vi "Brickbreaker.vi"() -> ()   [LabVIEW 2023]
uses:
  <vilib>/Utility/miscctls.llb/LVPositionTypeDef.ctl
panel:
  out "Brick":bool=TRUE
  out "Top":bool
  out "exit?":bool
  in  "STOP":bool
  out "BarPosition":T1
  out "BallPosition":T1
  out "Step":T1
  out "Score":i32
  out "Bar":bool
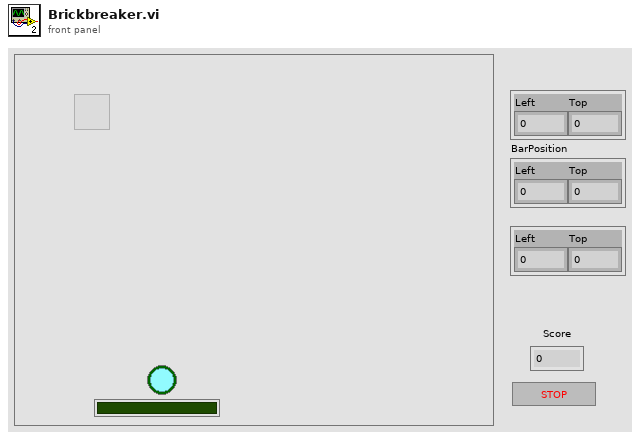
[diagram p1: front panel]
types:
  T1 = typedef "LVPositionTypeDef.ctl" = cluster{"Left":i32, "Top":i32}
  T2 = cluster{"BallPosition":T1, "Step":T1, "Score":i32, "BarPosition":T1, "BrickPosition":T1}
  T3 = typedef "eventvkey.ctl" = enum16{"ASCII", "Enter", "Return", "Shift", "Ctrl", "Alt", "Cmd", "Opt", "Caps", "NumLock", "Clear", "Break", "Up", "Down", "Left", "Right", "Insert", "Delete", "Home", "End", "PageUp", "PageDown", "Escape", "Help", "Pause", "ScrollLock", "F1", "F2", "F3", "F4", "F5", "F6", "F7", "F8", "F9", "F10", "F11", "F12", "F13", "F14", "F15", "F16", "F17", "F18", "F19", "F20", "F21", "F22", "F23", "F24", "Play", "VolumeUp", "VolumeDown", "Mute", "Two Byte Char"}
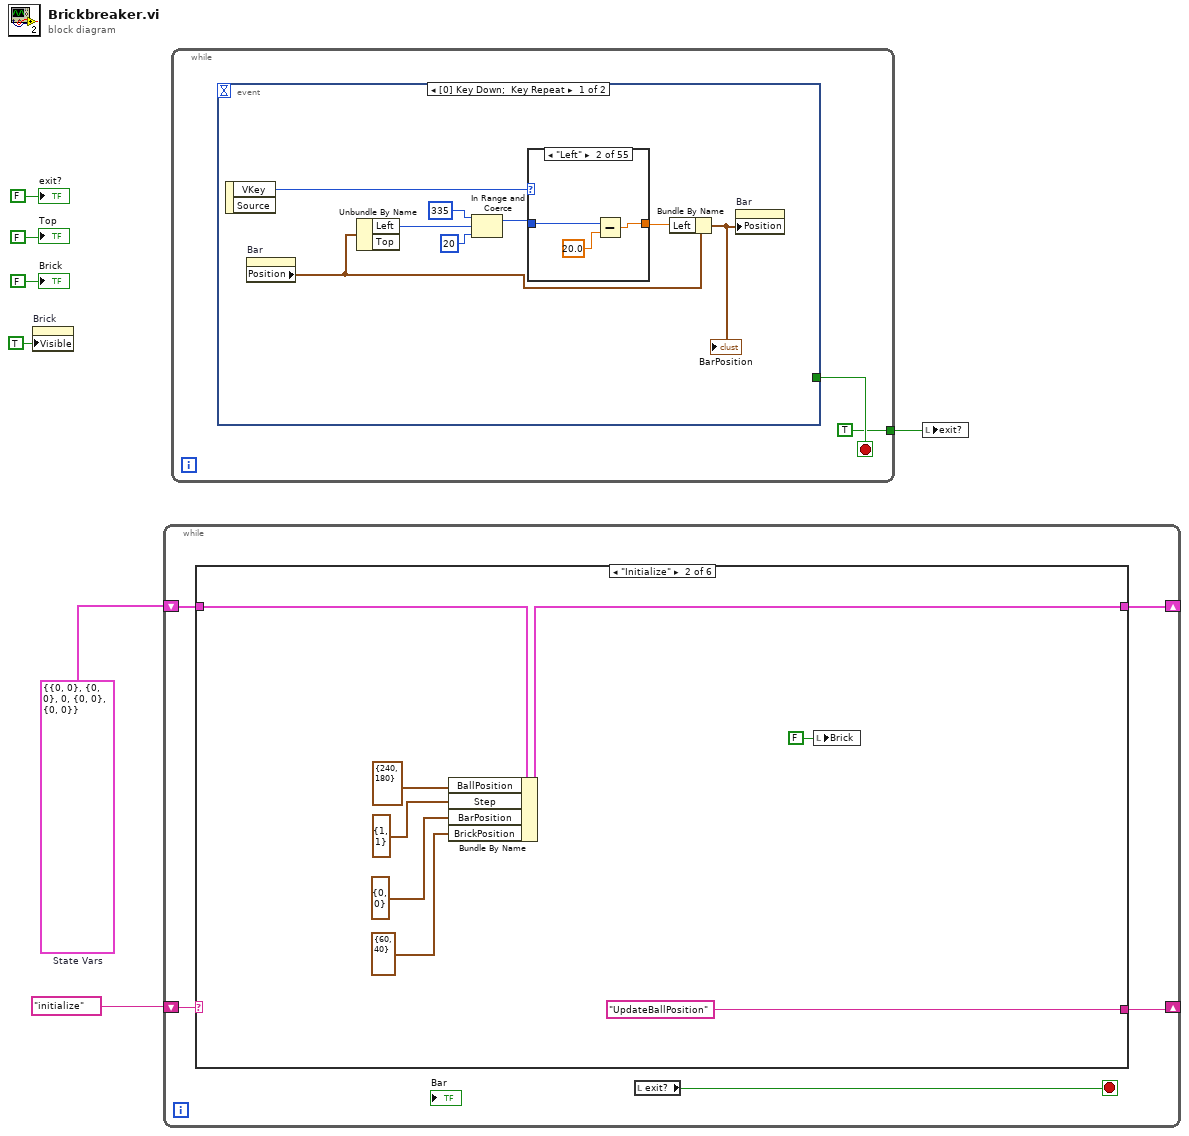
[diagram p0: block diagram]
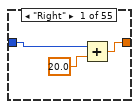
[diagram p2: hidden frame]
diagram:
  w6 = T2 {"BallPosition"={"Left"=0, "Top"=0}, "Step"={"Left"=0, "Top"=0}, "Score"=0, "BarPosition"={"Left"=0, "Top"=0}, "BrickPosition"={"Left"=0, "Top"=0}}  # State Vars
  n1 = property on="Brick" class="Bool"("Visible"=TRUE) -> ()  [unwired: 2 in, 2 out]
  n2 = while {
    shift-right: [w10] -> _
    shift-left: "initialize" -> [w9]
    shift-right: [w11] -> _
    shift-left: w6 -> [w12]
    stop <- w8 stop-if-true
    n3 = case shown="\"Initialize\"" w9 {
      selector: w9 -> [w13 _ _ _ _ _]
      tunnel: w12 -> [w14 w22 w32 w80 w100 w124]
      tunnel: [w14 w21 w51 w84 w101 w128] -> w11
      tunnel: [w13 "UpdateBallPosition" "BrickStep" "CheckPosition" "MoveBrick" "UpdateBallPosition"] -> w10
      frame "False", Default {
      }
      frame "Initialize" {
        n4 = Bundle By Name(cluster=w22, "BallPosition"=T1 {"Left"=240, "Top"=180} ("Position"), "Step"=T1 {"Left"=1, "Top"=1}, "BarPosition"=T1 {"Left"=0, "Top"=0}, "BrickPosition"=T1 {"Left"=60, "Top"=40}) -> (w21:T2)
        n5 = local write "Brick"(FALSE ("Brick")) -> ()
      }
      frame "CheckPosition" {
        n6 = Unbundle By Name(w32) -> ("BallPosition"=w61:T1, "Step"=w39:T1)
        n7 = Add(x=w61, y=w39) -> (x+y=w60:T1)
        n8 = property on="Bar" class="Bool (strict)"() -> ("Position"=w44:T1)  [unwired: 2 in, 2 out]
        n9 = Unbundle(w39) -> ("Left"=w53:i32, "Top"=w52:i32)
        n10 = Unbundle(w60) -> ("Left"=w59:i32, "Top"=w54:i32)
        n11 = property on="Top" class="Bool (strict)"() -> ("Position"=w43:T1)  [unwired: 2 in, 2 out]
        n12 = Unbundle By Name(w44) -> ("Left"=w45:i32, "Left"=w26:i32, "Top"=w28:i32)
        n13 = In Range and Coerce "xRange"(upper limit=460, x=w59, lower limit=0) -> (In Range?=w41:bool)  [unwired: 1 out]
        n14 = Unbundle By Name(w43) -> ("Left"=w27:i32, "Top"=w25:i32)
        n15 = In Range and Coerce "yRange"(upper limit=360, x=w54, lower limit=0) -> (coerced(x)=w49:i32, In Range?=w40:bool)
        n16 = Add(x=w45, y=120 ("x")) -> (x+y=w46:i32)
        n17 = Add(x=w25, y=12.0) -> (x+y=w23:dbl)
        n18 = In Range and Coerce(upper limit=w46, x=w27, lower limit=w26) -> (In Range?=w48:bool)  [unwired: 1 out]
        n19 = case shown="True" w41 {
          tunnel: [w76 w78] -> w37
          tunnel: w53 -> [w77 w78]
          frame False {
            n20 = Negate(x=w77) -> (-x=w76:i32)
          }
          frame True {
          }
        }
        n21 = case shown="True" w40 {
          tunnel: [w68 w73] -> w38
          tunnel: w52 -> [w67 w73]
          tunnel: w49 -> [_ w70]
          frame False {
            n22 = Negate(x=w67) -> (-x=w68:i32)
          }
          frame True {
            n23 = In Range and Coerce(upper limit=360, x=w70, lower limit=350) -> (In Range?=w69:bool)  [unwired: 1 out]
            n24 = case shown="False" w69 {
              frame False {
              }
              frame True {
                n25 = local write "exit?"(TRUE ("exit?")) -> ()
                n26 = One Button Dialog(message="Game Over") -> ()  [unwired: 1 in, 1 out]
              }
            }
          }
        }
        n27 = Equal?(x=w28, y=w23) -> (x = y?=w47:bool)
        n28 = And(x=w48, y=w47) -> (x .and. y?=w33:bool)
        n29 = case shown="True" w33 {
          tunnel: w38 -> [w62 w66]
          tunnel: w37 -> [w63 w64]
          tunnel: [w63 w64] -> w35
          tunnel: [w62 w65] -> w36
          frame False {
          }
          frame True {
            n30 = Negate(x=w66) -> (-x=w65:i32)
          }
        }
        n31 = Unbundle By Name(w32) -> ("BallPosition"=→"BallPosition":T1, "Step"=→"Step":T1, "Score"=→"Score":i32)
        n32 = Bundle("Left"=w35, "Top"=w36) -> (w34:cluster{"Left":i32, "Top":i32})  [unwired: 1 in]
        n33 = Bundle By Name(cluster=w32, "Step"=w34) -> (w51:T2)
      }
      frame "UpdateBallPosition" {
        n34 = Unbundle By Name(w80) -> ("BallPosition"=w85:T1, "Step"=w86:T1, "BrickPosition"=w79:T1)
        n35 = Add(x=w85, y=w86) -> (x+y=w83:T1)
        n36 = Bundle By Name(cluster=w80, "BrickPosition"=w79, "BallPosition"=w83) -> (w84:T2)
        n37 = property on="Brick" class="Bool"("Position"=w79) -> ()  [unwired: 2 in, 2 out]
        n38 = property on="Top" class="Bool (strict)"("Position"=w83) -> ()  [unwired: 2 in, 2 out]
        n39 = Wait (ms)(milliseconds to wait=u32 7) -> ()  [unwired: 1 out]
      }
      frame "BrickStep" {
        n40 = Unbundle By Name(w100) -> ("BallPosition"=w115:T1, "Step"=w114:T1)
        n41 = property on="Brick" class="Bool"() -> ("Position"=w113:T1)  [unwired: 2 in, 2 out]
        n42 = property on="Top" class="Bool (strict)"() -> ("Position"=w111:T1)  [unwired: 2 in, 2 out]
        n43 = Add(x=w115, y=w114) -> ()  [unwired: 1 out]
        n44 = property on="Brick" class="Bool"() -> ("Width"=w87:u32)  [unwired: 2 in, 2 out]
        n45 = property on="Brick" class="Bool"() -> ("Height"=w88:u32)  [unwired: 2 in, 2 out]
        n46 = Unbundle By Name(w111) -> ("Left"=w108:i32, "Top"=w109:i32)
        n47 = Unbundle By Name(w113) -> ("Left"=w112:i32, "Left"=w99:i32, "Top"=w110:i32, "Top"=w98:i32)
        n48 = Unbundle(w114) -> ("Left"=w107:i32, "Top"=w106:i32)
        n49 = Add(x=w109, y=12) -> (x+y=w95:i32)
        n50 = Add(x=w87, y=w112) -> (x+y=w97:u32)
        n51 = Add(x=w88, y=w110) -> (x+y=w96:u32)
        n52 = Add(x=w108, y=12) -> (x+y=w94:i32)
        n53 = In Range and Coerce(upper limit=w97, x=w94, lower limit=w99) -> (In Range?=w91:bool)  [unwired: 1 out]
        n54 = In Range and Coerce(upper limit=w96, x=w95, lower limit=w98) -> (In Range?=w90:bool)  [unwired: 1 out]
        n55 = And(x=w91, y=w90) -> (x .and. y?=w89:bool)
        n56 = case shown="True" w89 {
          tunnel: w107 -> [w118 w123]
          tunnel: w106 -> [w117 w122]
          tunnel: [w118 w121] -> w103
          tunnel: [w117 w120] -> w104
          frame False {
            n57 = local write "Brick"(FALSE ("Brick")) -> ()
          }
          frame True {
            n58 = Negate(x=w123) -> (-x=w121:i32)
            n59 = Negate(x=w122) -> (-x=w120:i32)
            n60 = local write "Brick"(TRUE ("Brick")) -> ()
          }
        }
        n61 = Bundle("Left"=w103, "Top"=w104) -> (w102:cluster{"Left":i32, "Top":i32})  [unwired: 1 in]
        n62 = Bundle By Name(cluster=w100, "Step"=w102) -> (w101:T2)
      }
      frame "MoveBrick" {
        n63 = property on="Brick" class="Bool"() -> ("Position"=w134:T1)  [unwired: 2 in, 2 out]
        n64 = Unbundle By Name(w134) -> ("Left"=w133:i32, "Top"=w132:i32)
        n65 = Unbundle By Name(w124) -> ("Score"=w126:i32)
        n66 = local read "Brick"() -> (w127:bool)
        n67 = case shown="False" w127 {
          tunnel: w133 -> [w138 _]
          tunnel: w132 -> [w137 _]
          tunnel: [w138 660 ("Left")] -> w131
          tunnel: [w137 0 ("Top")] -> w130
          tunnel: w126 -> [w136 w141]
          tunnel: [w136 w140] -> w125
          frame False {
          }
          frame True {
            n68 = property on="Brick" class="Bool"("Visible"=FALSE) -> ()  [unwired: 2 in, 2 out]
            n69 = Increment(x=w141) -> (x+1=w140:i32)
          }
        }
        n70 = Bundle("Left"=w131, "Top"=w130) -> (w129:cluster{"Left":i32, "Top":i32})  [unwired: 1 in]
        n71 = Bundle By Name(cluster=w124, "Score"=w125, "BrickPosition"=w129) -> (w128:T2)
        n72 = Unbundle By Name(w128) -> ()  [unwired: 1 out]
        n73 = property on="Brick" class="Bool"("Position"=w129) -> ()  [unwired: 2 in, 2 out]
      }
    }
    n74 = local read "exit?"() -> (w8:bool)
  }
  n75 = while {
    tunnel: [TRUE ("Top")] -> w3
    stop <- w145 stop-if-true
    n76 = event shown="[0] Key Down;  Key Repeat" {
      selector: _ -> [_ _]
      dyn-events: _ -> [_ _]
      timeout: _ -> [_ _]
      tunnel: [_ "STOP"] -> w145
      event Key Down; Key Repeat {
        n77 = event-data() -> ("VKey"=w146:T3)  [unwired: 1 in, 1 out]
        n78 = property on="Bar" class="Bool (strict)"() -> ("Position"=w152:T1)  [unwired: 2 in, 2 out]
        n79 = Unbundle By Name(w152) -> ("Left"=w149:i32)  [unwired: 1 out]
        n80 = In Range and Coerce(upper limit=335, x=w149, lower limit=20) -> (coerced(x)=w150:i32)  [unwired: 1 out]
        n81 = case shown="\"Left\"" w146 {
          tunnel: w150 -> [w155 w157 w160 w161 w162 w163 w164 w165 w166 w167 w168 w169 w170 w171 w172 w173 w174 w175 w176 w177 w178 w179 w180 w181 w182 w183 w184 w185 w186 w187 w188 w189 w190 w191 w192 w193 w194 w195 w196 w197 w198 w199 w200 w201 w202 w203 w204 w205 w206 w207 w208 w209 w210 w211 w212]
          tunnel: [w154 w158 w160 w161 w162 w163 w164 w165 w166 w167 w168 w169 w170 w171 w172 w173 w174 w175 w176 w177 w178 w179 w180 w181 w182 w183 w184 w185 w186 w187 w188 w189 w190 w191 w192 w193 w194 w195 w196 w197 w198 w199 w200 w201 w202 w203 w204 w205 w206 w207 w208 w209 w210 w211 w212] -> w153
          frame "Right" {
            n82 = Add(x=w155, y=20.0) -> (x+y=w154:dbl)
          }
          frame "Left" {
            n83 = Subtract(x=w157, y=20.0) -> (x-y=w158:dbl)
          }
          frame "F16" {
          }
          frame "F17" {
          }
          frame "F18" {
          }
          frame "F19" {
          }
          frame "F20" {
          }
          frame "F21" {
          }
          frame "F22" {
          }
          frame "F23" {
          }
          frame "F24" {
          }
          frame "Play" {
          }
          frame "VolumeUp" {
          }
          frame "VolumeDown" {
          }
          frame "Mute" {
          }
          frame "Two Byte Char" {
          }
          frame "Insert" {
          }
          frame "Delete" {
          }
          frame "Home" {
          }
          frame "End" {
          }
          frame "PageUp" {
          }
          frame "PageDown" {
          }
          frame "Escape" {
          }
          frame "Help" {
          }
          frame "Pause" {
          }
          frame "ScrollLock" {
          }
          frame "F1" {
          }
          frame "F2" {
          }
          frame "F3" {
          }
          frame "F4" {
          }
          frame "F5" {
          }
          frame "F6" {
          }
          frame "F7" {
          }
          frame "F8" {
          }
          frame "F9" {
          }
          frame "F10" {
          }
          frame "F11" {
          }
          frame "F12" {
          }
          frame "F13" {
          }
          frame "F14" {
          }
          frame "F15" {
          }
          frame "Down" {
          }
          frame "Up" {
          }
          frame "Break" {
          }
          frame "Clear" {
          }
          frame "NumLock" {
          }
          frame "Caps" {
          }
          frame "Opt" {
          }
          frame "Cmd" {
          }
          frame "Alt" {
          }
          frame "Ctrl" {
          }
          frame "Shift" {
          }
          frame "Return" {
          }
          frame "Enter" {
          }
          frame "ASCII" {
          }
        }
        n84 = Bundle By Name(cluster=w152, "Left"=w153) -> (w151:T1)
        "BarPosition" <- w151
        n85 = property on="Bar" class="Bool (strict)"("Position"=w151) -> ()  [unwired: 2 in, 2 out]
      }
      event "STOP": Value Change {
        n86 = event-data() -> ()  [unwired: 1 in, 4 out]
      }
    }
  }
  n87 = local write "exit?"(w3) -> ()
  "exit?" <- FALSE ("exit?")
  "Top" <- FALSE ("Top")
  "Brick" <- FALSE ("Brick")
